vi "Teleop.vi"(10 "Match Info":T1={"Autonomous Elapsed Seconds"=0.0, "TeleOp Elapsed Seconds"=0.0, "Disabled Elapsed Seconds"=0.0, "Visited Autonomous"=FALSE, "Visited TeleOp"=FALSE, "Visited Disabled"=FALSE, "Autonomous Settings"={"Autonomous Style"=enum."Independent", "VI Refnum"=refnum}}, 11 "Call Context":T2) -> ()   [LabVIEW 2017]
doc: "This VI is called for each TeleOp packet received from the DS where the robot is not disabled. It is often used to read from the joysticks and update I/O or to update setpoints for timed control loops. It should complete and return within 20 milliseconds or it may miss DS packets."
uses:
  <vilib>/Rock Robotics/WPI/DriverStation/WPI_DriverStationDerivedRobotMode.ctl
  <vilib>/Rock Robotics/WPI/DriverStation/WPI_DriverStationMatch Info.ctl
  Public/Documents/Cross The Road Electronics/Phoenix-LabVIEW/CANifier/CTRE_CANifier_PWMChannel.ctl
  Public/Documents/Cross The Road Electronics/Phoenix-LabVIEW/CANifier/CTRE_CANifier_LEDChannel.ctl
  <vilib>/Rock Robotics/WPI/Utilities/WPI_GetSetVariantRefNum.vi
  Robot Global Data.vi
  <vilib>/gmath/NI_Gmath.lvlib
panel:
  in  "Duty cycles and Periods":dbl[][](array[numeric])
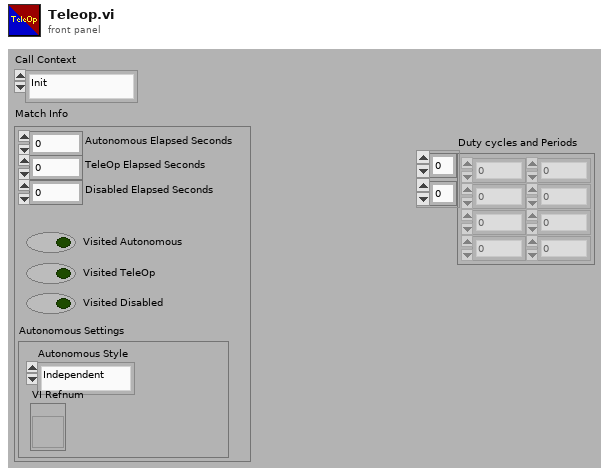
[diagram p1: front panel]
types:
  T1 = typedef "WPI_DriverStationMatch Info.ctl" = cluster{"Autonomous Elapsed Seconds":dbl, "TeleOp Elapsed Seconds":dbl, "Disabled Elapsed Seconds":dbl, "Visited Autonomous":bool, "Visited TeleOp":bool, "Visited Disabled":bool, "Autonomous Settings":cluster{"Autonomous Style":enum16{"Iterative", "Independent"}, "VI Refnum":refnum<vi>}}
  T2 = typedef "WPI_DriverStationDerivedRobotMode.ctl" = enum16{"Init", "Execute", "Stop"}
  T3 = typedef "CTRE_CANifier_PWMChannel.ctl" = enum16{"PWMChannel0", "PWMChannel1", "PWMChannel2", "PWMChannel3"}
  T4 = typedef "CTRE_CANifier_LEDChannel.ctl" = enum32{"LEDChannelA", "LEDChannelB", "LEDChannelC"}
  T5 = typedef "CTRE_CANifier_DeviceRef.ctl" = cluster{"DeviceStatus":errorcluster, "Device Number":u8, "Handle":u64, "UsageFrame":u32, "Library Path":path}
  T6 = typedef "WPI_JoystickDevRef.ctl" = cluster{"Device":T7}
  T7 = typedef "WPI_JoystickDeviceEnum.ctl" = enum16{"USB 0", "USB 1", "USB 2", "USB 3", "USB 4", "USB 5"}
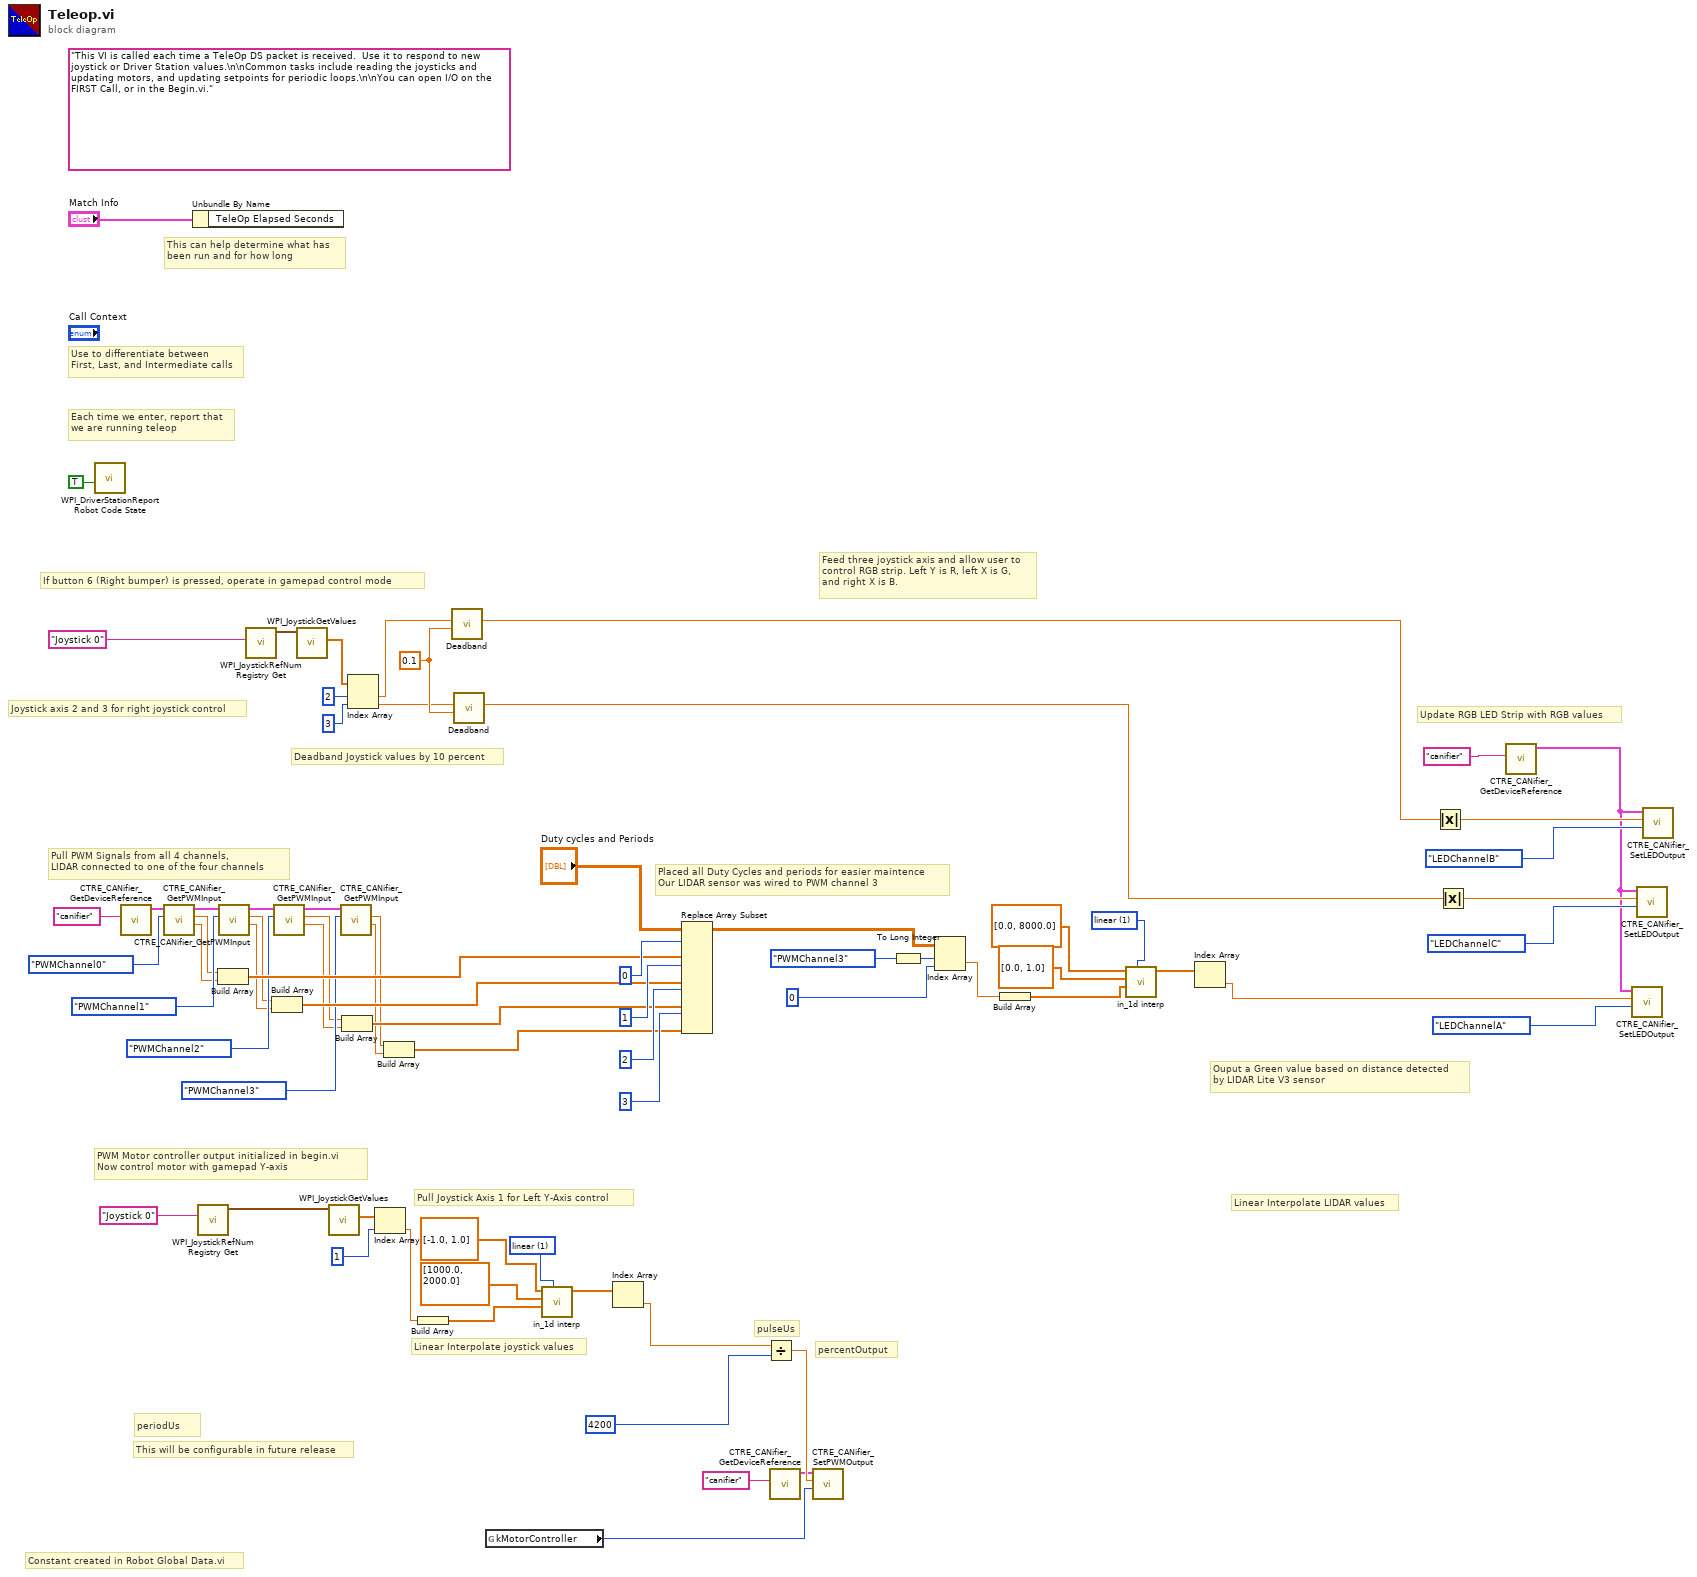
[diagram p0: block diagram]
diagram:
  w32 = 1 items=["nearest", "linear", "spline", "cubic Hermite", "Lagrange"] ("method")
  w45 = 1 items=["nearest", "linear", "spline", "cubic Hermite", "Lagrange"] ("method")
  w70 = 0.1
  (unwired) "This VI is called each time a TeleOp DS packet is received.  Use it to respond to new joystick or Driver Station values.\n\nCommon tasks include reading the joysticks and updating motors, and updating setpoints for periodic loops.\n\nYou can open I/O on the FIRST Call, or in the Begin.vi."
  # "Pull PWM Signals from all 4 channels, \nLIDAR connected to one of the four channels"
  # "Update RGB LED Strip with RGB values"
  # "Pull Joystick Axis 1 for Left Y-Axis control"
  # "Linear Interpolate joystick values"
  # "Constant created in Robot Global Data.vi"
  # "This will be configurable in future release"
  # "percentOutput"
  # "periodUs"
  # "pulseUs"
  # "PWM Motor controller output initialized in begin.vi\nNow control motor with gamepad Y-axis"
  # "Joystick axis 2 and 3 for right joystick control"
  # "Placed all Duty Cycles and periods for easier maintence\nOur LIDAR sensor was wired to PWM channel 3"
  # "Ouput a Green value based on distance detected\nby LIDAR Lite V3 sensor"
  # "Linear Interpolate LIDAR values"
  # "If button 6 (Right bumper) is pressed, operate in gamepad control mode"
  # "Deadband Joystick values by 10 percent"
  # "Feed three joystick axis and allow user to\ncontrol RGB strip. Left Y is R, left X is G, \nand right X is B."
  # "Each time we enter, report that\nwe are running teleop"
  # "Use to differentiate between\nFirst, Last, and Intermediate calls"
  # "This can help determine what has\nbeen run and for how long"
  n1 = call <vilib>:"WPI_DriverStationReport Robot Code State.vi"("TeleOp"=TRUE ("Autonomous")) -> ()  [unwired: 10 in, 1 out]
  n2 = call "CTRE_CANifier_GetDeviceReference.vi"("refnum name"="canifier") -> ("CANifierDevRef"=w16:T5)  [unwired: 9 in, 1 out]
  n3 = call "CTRE_CANifier_GetPWMInput.vi"("PWMChannel"=CTRE_CANifier_PWMChannel."PWMChannel0", "CANifierDevRef"=w16) -> ("Period"=w7:sgl, "Duty Cycle"=w8:sgl, "CANifierDevRef"=w9:T5)  [unwired: 6 in, 1 out]
  n4 = Unbundle By Name("Match Info") -> ()  [unwired: 1 out]
  n5 = call <vilib>:"WPI_JoystickRefNum Registry Get.vi"("refnum name"="Joystick 0") -> ("JoystickDevRef"=w39:T6)  [unwired: 9 in, 1 out]
  n6 = Build Array(w8, w7) -> (w62:sgl[])
  n7 = call "CTRE_CANifier_GetPWMInput.vi"("PWMChannel"=CTRE_CANifier_PWMChannel."PWMChannel1", "CANifierDevRef"=w9) -> ("Period"=w4:sgl, "Duty Cycle"=w5:sgl, "CANifierDevRef"=w10:T5)  [unwired: 6 in, 1 out]
  n8 = call <vilib>:"WPI_JoystickRefNum Registry Get.vi"("refnum name"="Joystick 0") -> ("JoystickDevRef"=w68:T6)  [unwired: 1 in, 9 out]
  n9 = Build Array(w5, w4) -> (w61:sgl[])
  n10 = call "CTRE_CANifier_GetPWMInput.vi"("PWMChannel"=CTRE_CANifier_PWMChannel."PWMChannel2", "CANifierDevRef"=w10) -> ("Period"=w3:sgl, "Duty Cycle"=w6:sgl, "CANifierDevRef"=w11:T5)  [unwired: 6 in, 1 out]
  n11 = call <vilib>:"WPI_JoystickGetValues.vi"("JoystickDevRef"=w68) -> ("Axes"=w69:dbl[])  [unwired: 6 in, 4 out]
  n12 = call <vilib>:"WPI_JoystickGetValues.vi"("JoystickDevRef"=w39) -> ("Axes"=w38:dbl[])  [unwired: 6 in, 4 out]
  n13 = call "CTRE_CANifier_GetPWMInput.vi"("PWMChannel"=CTRE_CANifier_PWMChannel."PWMChannel3", "CANifierDevRef"=w11) -> ("Period"=w1:sgl, "Duty Cycle"=w2:sgl)  [unwired: 6 in, 2 out]
  n14 = Build Array(w6, w3) -> (w60:sgl[])
  n15 = Index Array(array=w69, index #1=2, index #2=3) -> (element #1=w52:dbl, element #2=w53:dbl)
  n16 = Index Array(array=w38, index=1) -> (element=w34:dbl)
  n17 = Build Array(w2, w1) -> (w59:sgl[])
  n18 = Build Array(w34) -> (w28:dbl[])
  n19 = call "Deadband.vi"("deadband"=w70, "value"=w52) -> ("ret value"=w48:dbl)  [unwired: 9 in]
  n20 = call "Deadband.vi"("deadband"=w70, "value"=w53) -> ("ret value"=w49:dbl)  [unwired: 9 in]
  n21 = global read "Robot Global Data.vi" "kMotorController"() -> (w18:T3)
  n22 = call <vilib>:"in_1d interp.vi"("method"=w32, "xi"=w28, "Y"=dbl[] [1000.0, 2000.0], "X"=dbl[] [-1.0, 1.0]) -> ("yi"=w31:dbl[])  [unwired: 6 in, 1 out]
  n23 = Index Array(array=w31) -> (element=w33:dbl)  [unwired: 1 in]
  n24 = Replace Array Subset(array="Duty cycles and Periods", new element #1=w62, index (row) #1=0, new element #2=w61, index (row) #2=1, new element #3=w60, index (row) #3=2, new element #4=w59, index (row) #4=3) -> (w54:dbl[][])  [unwired: 4 in]
  n25 = Divide(x=w33, y=4200) -> (x/y=w36:dbl)
  n26 = call "CTRE_CANifier_GetDeviceReference.vi"("refnum name"="canifier") -> ("CANifierDevRef"=w19:T5)  [unwired: 9 in, 1 out]
  n27 = call "CTRE_CANifier_SetPWMOutput.vi"("PWMChannel"=w18, "Duty Cycle"=w36, "CANifierDevRef"=w19) -> ()  [unwired: 7 in, 2 out]
  n28 = To Long Integer(number=CTRE_CANifier_PWMChannel."PWMChannel3" ("PWMChannel")) -> (32bit integer=w56:i32)
  n29 = Index Array(array=w54, index (row)=w56, index (col)=0) -> (element=w47:dbl)
  n30 = Build Array(w47) -> (w42:dbl[])
  n31 = call <vilib>:"in_1d interp.vi"("method"=w45, "xi"=w42, "Y"=dbl[] [0.0, 1.0], "X"=dbl[] [0.0, 8000.0]) -> ("yi"=w41:dbl[])  [unwired: 6 in, 1 out]
  n32 = Index Array(array=w41) -> (element=w46:dbl)  [unwired: 1 in]
  n33 = Absolute Value(x=w48) -> (abs(x)=w23:dbl)
  n34 = Absolute Value(x=w49) -> (abs(x)=w24:dbl)
  n35 = call "CTRE_CANifier_GetDeviceReference.vi"("refnum name"="canifier") -> ("CANifierDevRef"=w21:T5)  [unwired: 9 in, 1 out]
  n36 = call "CTRE_CANifier_SetLEDOutput.vi"("LEDChannel"=CTRE_CANifier_LEDChannel."LEDChannelA", "Percent Output"=w46, "CANifierDevRef"=w21) -> ()  [unwired: 7 in, 2 out]
  n37 = call "CTRE_CANifier_SetLEDOutput.vi"("LEDChannel"=CTRE_CANifier_LEDChannel."LEDChannelC", "Percent Output"=w24, "CANifierDevRef"=w21) -> ()  [unwired: 7 in, 2 out]
  n38 = call "CTRE_CANifier_SetLEDOutput.vi"("LEDChannel"=CTRE_CANifier_LEDChannel."LEDChannelB", "Percent Output"=w23, "CANifierDevRef"=w21) -> ()  [unwired: 7 in, 2 out]
